vi "Identify.vi"(8 "error in (no error)":errorcluster, 11 "PSU in":refnum<class "Power Supply Parent.lvclass">) -> (0 "error out":errorcluster, 2 "Identification":string, 3 "PSU out":refnum<class "Power Supply Parent.lvclass">)   [LabVIEW 2017, in "Power Supply Driver.lvlib" / "Power Supply Parent.lvclass"]
uses:
  Power Supply Parent.lvclass
  <vilib>/Utility/error.llb/Error Cluster From Error Code.vi
  <vilib>/ErrorRing/Error Ring.xnode
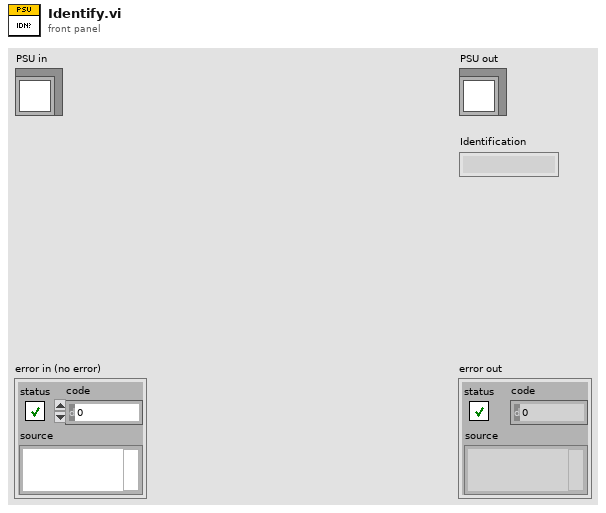
[diagram p1: front panel]
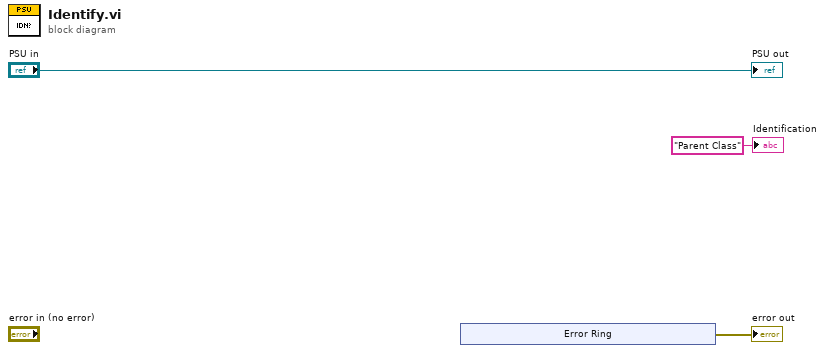
[diagram p0: block diagram]
diagram:
  n1 = xnode "Error Ring"() -> ("error out"=→"error out":errorcluster)
  "PSU out" <- "PSU in"
  "Identification" <- "Parent Class" ("Identification")
